vi "MainVI.vi"() -> ()   [LabVIEW 2022 SP3]
uses:
  <vilib>/measure/madcrms.llb/Basic Averaged DC-RMS for N Chan.vi
  <vilib>/express/express analysis/Spectral/Block/exnSpectralBlock spectral measurements RMS poly.vi
  <vilib>/express/express analysis/Spectral/Block/exnSpectralBlock spectral measurements RMS DDT.vi
  <vilib>/xnet/xnet.llb/XNET Write (Signal Single-point).vi
  <vilib>/xnet/xnet.llb/XNET Read (Signal Single-point).vi
  <vilib>/express/express analysis/Spectral/XNode/ExpressSpectralMeasurementsBlockNode.xnode
  <vilib>/measure/NI_MAPro.lvlib
panel:
  out "DAQmx error":errorcluster
  out "Unfiltered Current Spectrograph":dynamicdata(graph)
  out "Unfiltered Voltage Spectrograph":dynamicdata(graph)
  out "Filtered Current Spectrograph":dynamicdata(graph)
  out "Filtered Voltage Spectrograph":dynamicdata(graph)
  out "Unfiltered Voltage":dynamicdata(graph)
  out "Unfiltered Current":dynamicdata(graph)
  out "Filtered Current":dynamicdata(graph) caption="Filtered Signal"
  out "Filtered Voltage":dynamicdata(graph) caption="Filtered Signal"
  out "X1 Current":dbl
  out "X2 Current":dbl
  out "X3 Current":dbl
  out "X2 Voltage":dbl
  out "X3 Voltage":dbl
  out "X1 Votage":dbl
  in  "Stop":bool
  in  "Voltage LPF cutoff":dbl=200.0 caption="Lower Cut-Off"
  in  "Current LPF Cutoff":dbl=200.0 caption="Lower Cut-Off"
  out "AC Current":dbl
  out "AC Voltage":dbl
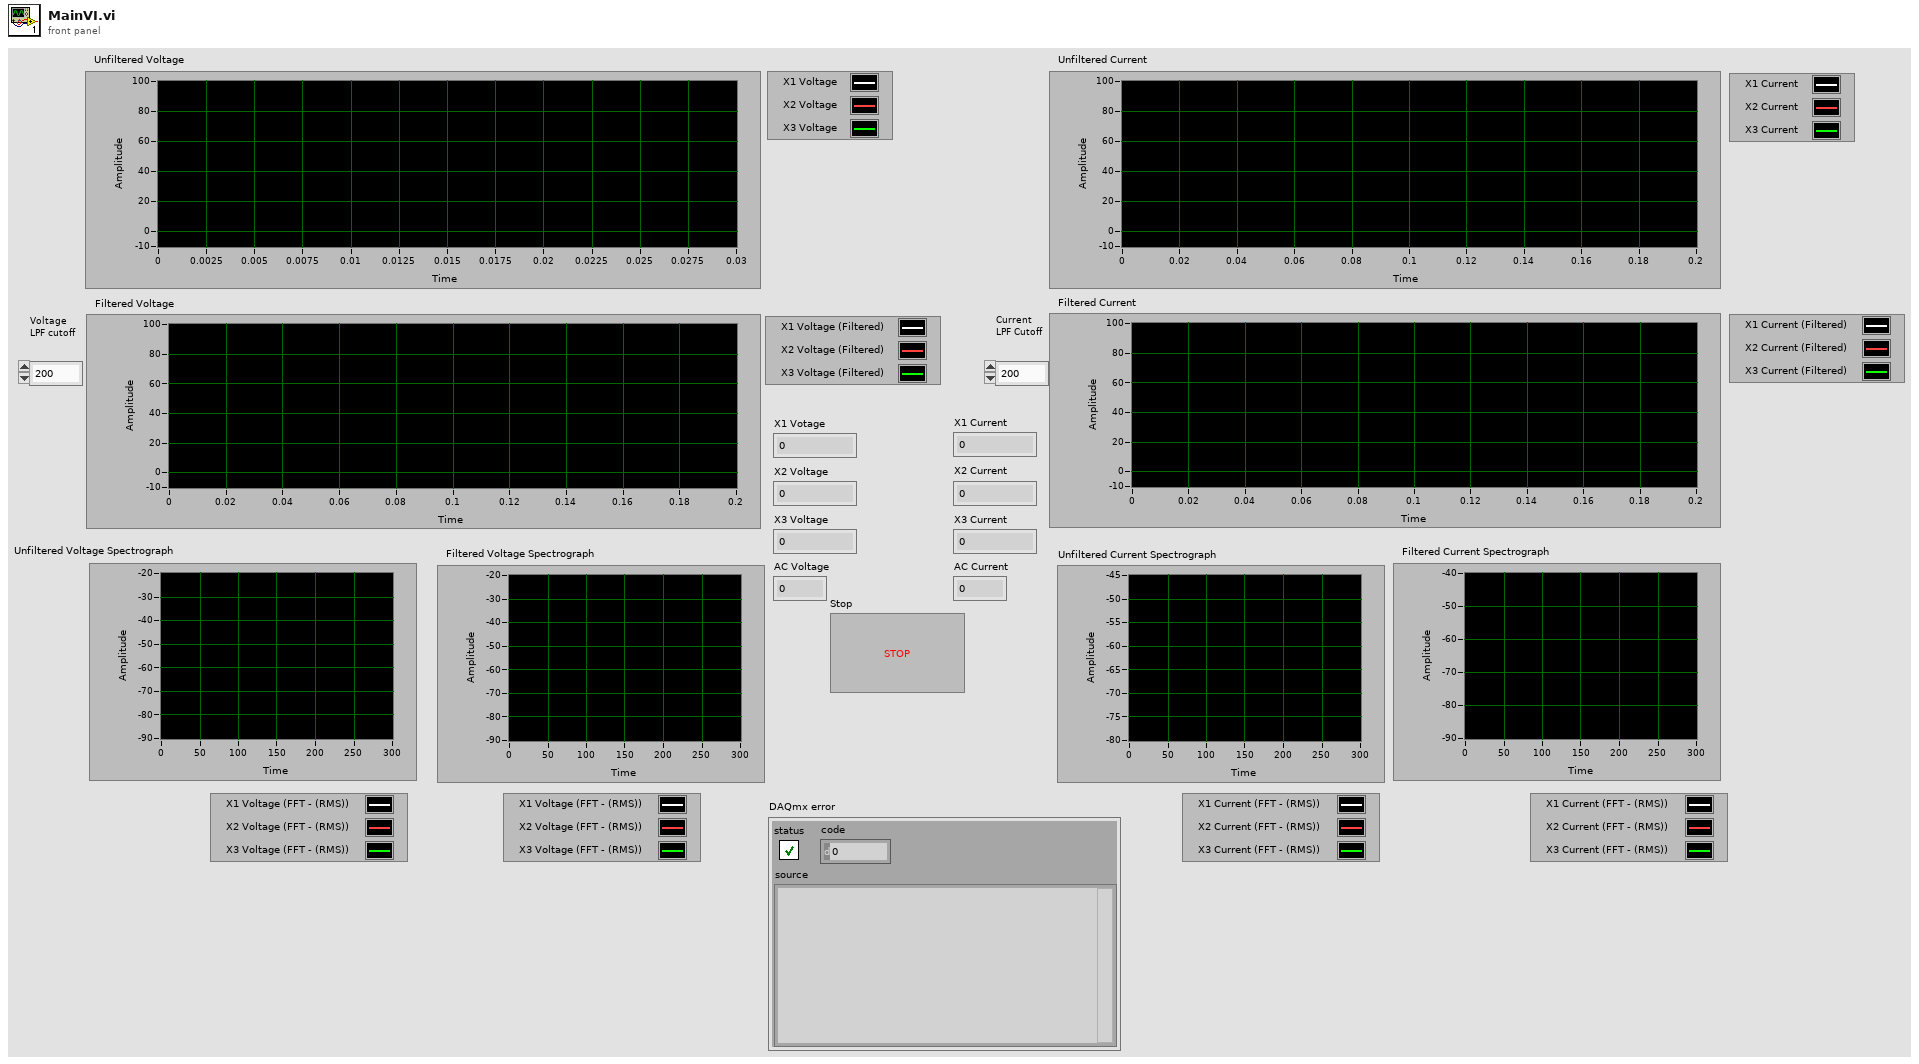
[diagram p1: front panel]
types:
  T1 = cluster{"averaging mode":u16, "weighting mode":u16, "number of averages":u32}
  T2 = cluster{"dB On (F)":bool, "unwrap phase (F)":bool, "convert to degree (F)":bool}
  T3 = cluster{"RMS values[0]":dbl, "RMS values[1]":dbl, "RMS values[2]":dbl}
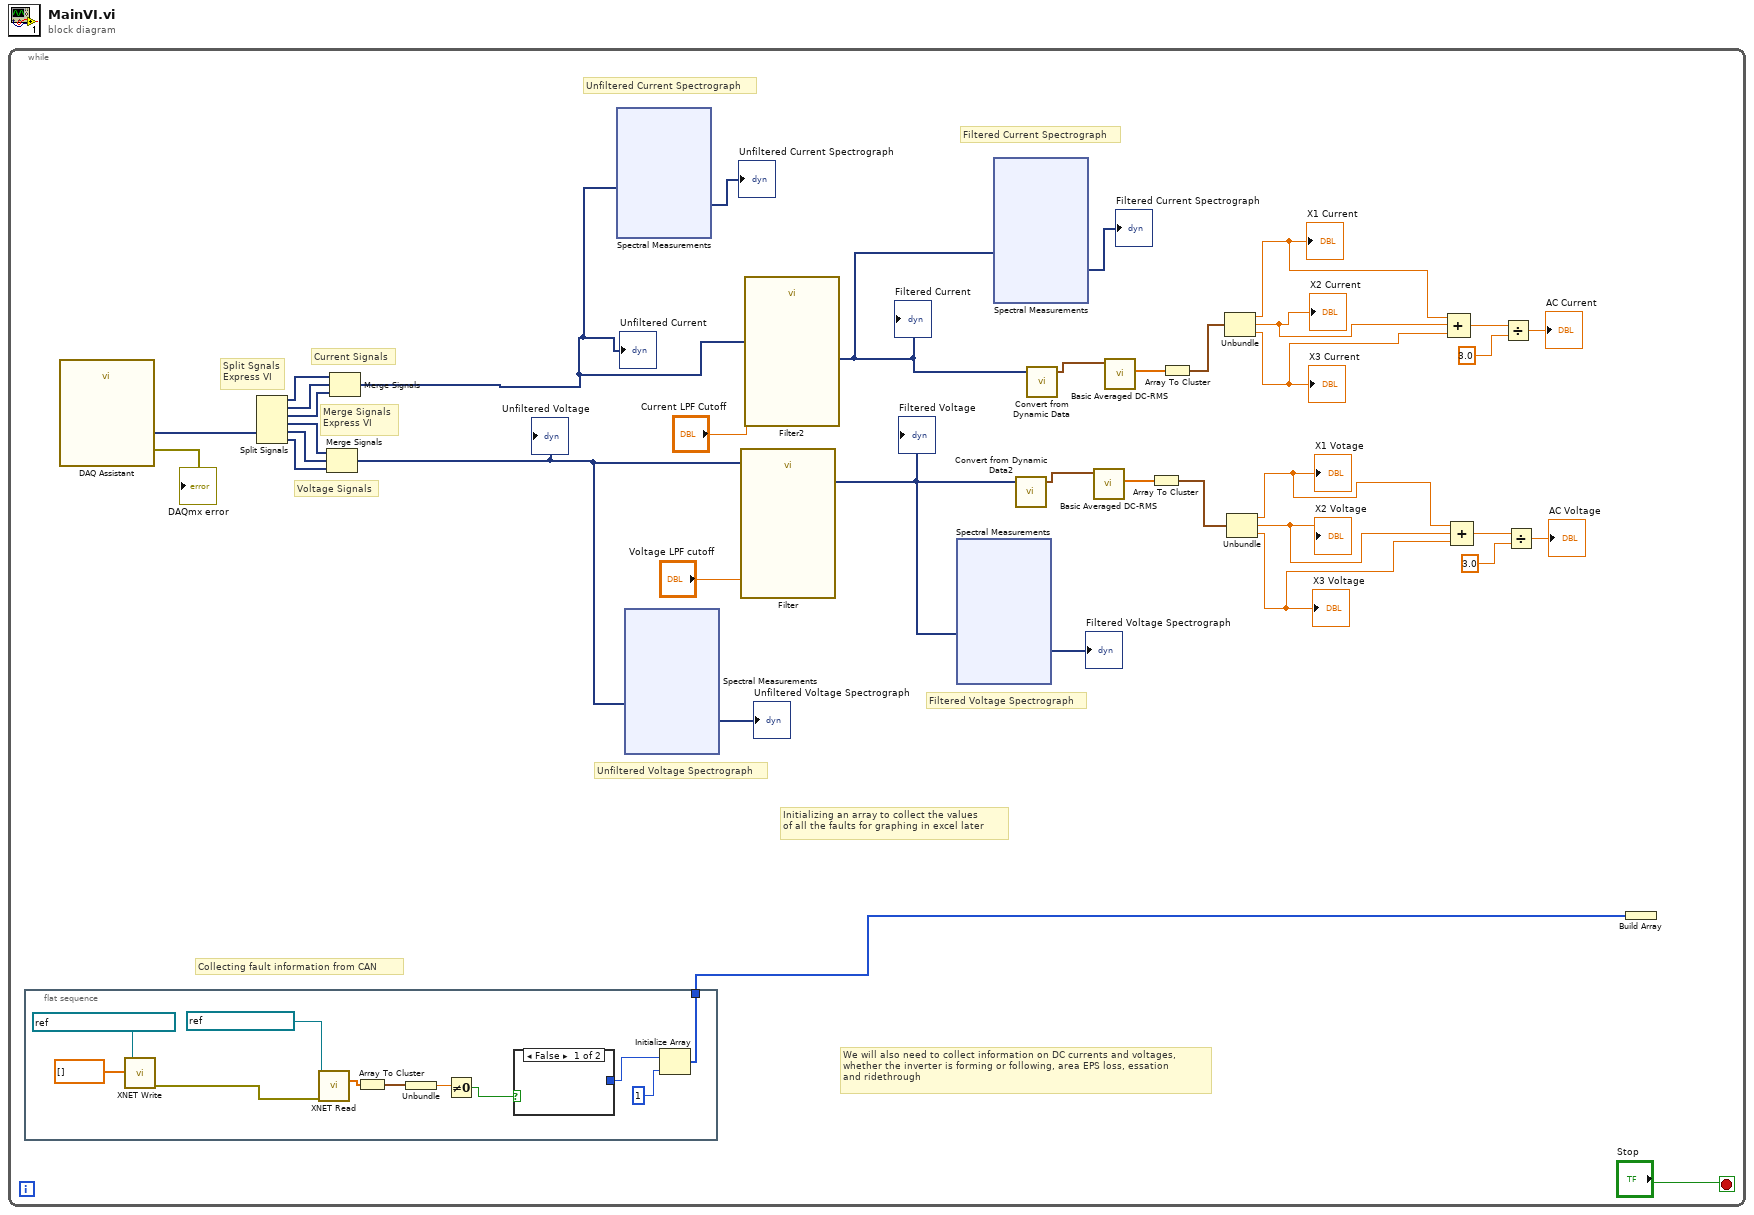
[diagram p0: block diagram]
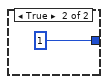
[diagram p2: hidden frame]
diagram:
  n1 = while {
    stop <- "Stop" stop-if-true
    # "We will also need to collect information on DC currents and voltages, \nwhether the inverter is forming or following, area EPS loss, essation \nand ridethrough"
    # "Collecting fault information from CAN"
    # "Initializing an array to collect the values \nof all the faults for graphing in excel later"
    # "Filtered Voltage Spectrograph"
    # "Filtered Current Spectrograph"
    # "Unfiltered Voltage Spectrograph"
    # "Unfiltered Current Spectrograph"
    # "Merge Signals\nExpress VI"
    # "Split Sgnals\nExpress VI"
    # "Voltage Signals"
    # "Current Signals"
    n2 = flat-sequence {
      tunnel: [w40] -> w1
      frame #0 {
        n3 = call-poly <vilib>:"XNET Write.vi"("session in"=refnum<k21> "ParameterQuery_Mux", "data"=dbl[] []) -> ("error out"=w46:errorcluster)  [unwired: 12 in, 1 out]
        n4 = call-poly <vilib>:"XNET Read.vi"("session in"=refnum<k21> "General_Fault", "error in (no error)"=w46) -> ("data"=w45:dbl[])  [unwired: 11 in, 2 out]
        n5 = Array To Cluster(array=w45) -> (cluster=w44:cluster{"data[0]":dbl})
        n6 = Unbundle(w44) -> ("data[0]"=w43:dbl)
        n7 = Not Equal To 0?(x=w43) -> (x != 0?=w42:bool)
        n8 = case shown="False" w42 {
          tunnel: [_ 1] -> w41
          frame False {
          }
          frame True {
          }
        }
        n9 = Initialize Array(w41, 1 ("dimension size")) -> (w40:i32[])
      }
    }
    n10 = call "DAQ Assistant"() -> ("data"=w36:dynamicdata, "error out"=→"DAQmx error":errorcluster)  [unwired: 16 in, 2 out]
    n11 = Split Signals(w36) -> (w15:dynamicdata, w16:dynamicdata, w17:dynamicdata, w35:dynamicdata, w34:dynamicdata, w33:dynamicdata)  [unwired: 6 in]
    n12 = Merge Signals(w35, w34, w33) -> (w31:dynamicdata)
    "Unfiltered Voltage" <- w31
    n13 = Merge Signals(w15, w16, w17) -> (w8:dynamicdata)
    "Unfiltered Current" <- w8
    n14 = xnode "Spectral Measurements"("Signals"=w8) -> ("FFT - (RMS)"=→"Unfiltered Current Spectrograph":dynamicdata)  [unwired: 1 in, 2 out]
    n15 = xnode "Spectral Measurements"("Signals"=w31) -> ("FFT - (RMS)"=→"Unfiltered Voltage Spectrograph":dynamicdata)  [unwired: 1 in, 2 out]
    n16 = call "Filter"("Lower Cut-Off"="Voltage LPF cutoff", "Signal"=w31) -> ("Filtered Signal"=w21:dynamicdata)  [unwired: 8 in, 1 out]
    "Filtered Voltage" <- w21
    n17 = call "Filter2"("Lower Cut-Off"="Current LPF Cutoff", "Signal"=w8) -> ("Filtered Signal"=w28:dynamicdata)  [unwired: 8 in, 1 out]
    "Filtered Current" <- w28
    n18 = xnode "Spectral Measurements"("Signals"=w21) -> ("FFT - (RMS)"=→"Filtered Voltage Spectrograph":dynamicdata)  [unwired: 1 in, 2 out]
    n19 = xnode "Spectral Measurements"("Signals"=w28) -> ("FFT - (RMS)"=→"Filtered Current Spectrograph":dynamicdata)  [unwired: 1 in, 2 out]
    n20 = call "Convert from Dynamic Data2"("Dynamic Data Type"=w21) -> ("Array of Waveform"=w22:waveform(dbl)[])  [unwired: 3 in]
    n21 = call "Convert from Dynamic Data"("Dynamic Data Type"=w28) -> ("Array of Waveform"=w27:waveform(dbl)[])  [unwired: 3 in]
    n22 = call-poly <vilib>:"Basic Averaged DC-RMS.vi"("signals in"=w22) -> ("RMS values"=w23:dbl[])  [unwired: 7 in, 3 out]
    n23 = call-poly <vilib>:"Basic Averaged DC-RMS.vi"("signals in"=w27) -> ("RMS values"=w26:dbl[])  [unwired: 7 in, 3 out]
    n24 = Array To Cluster(array=w23) -> (cluster=w24:T3)
    n25 = Array To Cluster(array=w26) -> (cluster=w25:T3)
    n26 = Unbundle(w25) -> ("RMS values[0]"=w14:dbl, "RMS values[1]"=w13:dbl, "RMS values[2]"=w12:dbl)
    "X1 Current" <- w14
    "X2 Current" <- w13
    "X3 Current" <- w12
    n27 = Unbundle(w24) -> ("RMS values[0]"=w4:dbl, "RMS values[1]"=w3:dbl, "RMS values[2]"=w2:dbl)
    "X2 Voltage" <- w3
    "X3 Voltage" <- w2
    "X1 Votage" <- w4
    n28 = Compound Arithmetic op=ADD(w14, w13, w12) -> (w11:dbl)
    n29 = Compound Arithmetic op=ADD(w4, w3, w2) -> (w5:dbl)
    n30 = Divide(x=w11, y=3.0) -> (x/y=→"AC Current":dbl)
    n31 = Divide(x=w5, y=3.0) -> (x/y=→"AC Voltage":dbl)
    n32 = Build Array(w1) -> ()  [unwired: 1 out]
  }
